vi "sender.vi"() -> ()   [LabVIEW 2009]
uses:
  Robot Status.ctl
  <vilib>/Platform/TimedLoop/XDataNode/XDataNode.xnode
  <vilib>/Platform/TimedLoop/XDataNode/loadlvalarms.vi
  <vilib>/Platform/TimedLoop/XDataNode/timing_clust.ctl
  <vilib>/Platform/TimedLoop/XDataNode/nitl_modes.ctl
  <vilib>/Platform/TimedLoop/XDataNode/wakeup.ctl
  UDP Lib/UDP Network Location.ctl
  cRIO/Functional Global Variables/Actions for FG's.ctl
  <vilib>/Platform/TimedLoop/XDataNode/XDNodeRunTimeDep.lvlib
panel:
  out "Status out":T1
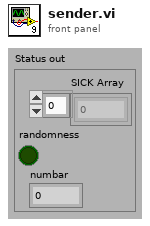
[diagram p1: front panel]
types:
  T1 = typedef "Robot Status.ctl" = cluster{"SICK Array":dbl[], "randomness":bool, "numbar":dbl}
  T2 = typedef "UDP Base.ctl" = cluster{"UDP Session":refnum<k16>, "UDP Socket Params":T3}
  T3 = typedef "UDP Socket Params.ctl" = cluster{"Local Port":u16, "Read Timeout":i32, "Write Timeout":i32}
  T4 = typedef "XDNodeRunTimeDep.lvlib/timing_clust.ctl" = cluster{"Expected End [f-1]":u64, "Actual End [f-1]":u64, "Finished Late? [f-1]":bool, "Expected End [i-1]":u64, "Actual End [i-1]":u64, "Finished Late? [i-1]":bool, "Expected Start [i]":u64, "Actual Start [i]":u64, "Expected Start [f]":u64, "Actual Start [f]":u64, "Source Name":string, "Structure Name":string, "Period":i64, "Deadline":i64, "Offset":i64, "Start":i64, "Priority":i32, "Timeout":i32, "Mode":T5, "Wakeup Reason":T6, "Error":errorcluster, "Source Type":string, "Secondary Source Type":string, "Global End Time":u64, "Global Start Time":u64, "Frame Duration":u64, "Iteration Duration":u64, "Assigned CPU":i32, "I/O Scan Engine Mode":u32}
  T5 = typedef "XDNodeRunTimeDep.lvlib/nitl_modes.ctl" = enum32{"No Change", "Process missed periods, maintain original phase", "Discard missed periods, maintain original phase", "Process missed periods, ignore original phase", "Discard missed periods, ignore original phase"}
  T6 = typedef "XDNodeRunTimeDep.lvlib/wakeup.ctl" = enum32{"Normal", "Aborted", "Asynchronous wakeup", "Timing source error", "Timed loop error", "Timeout"}
  T7 = typedef "UDP Network Location.ctl" = cluster{"IP Address":string, "Port":u16}
  T8 = typedef "Actions for FG's.ctl" = enum16{"Read", "Write"}
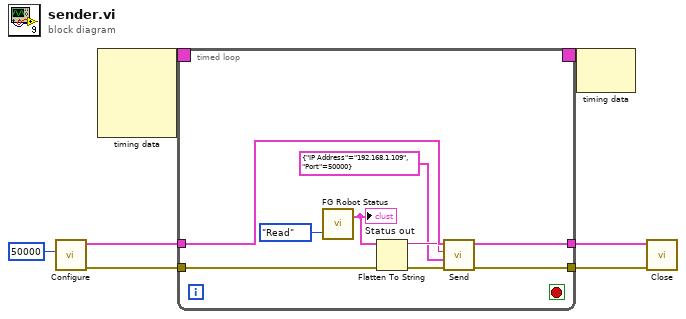
[diagram p0: block diagram]
diagram:
  n1 = call "Configure.vi"("Local Port"=u16 50000) -> ("error out"=w2:errorcluster, "UDP Base out"=w3:T2)  [unwired: 9 in]
  n2 = node-c288() -> (w7:T4)  [unwired: 4 in]
  n3 = timed-loop {
    timing: w7 -> [_]
    timing-out: [_] -> w6
    tunnel: [w15] -> w5
    tunnel: [w14] -> w4
    tunnel: w3 -> [w13]
    tunnel: w2 -> [w10]
    stop <- _ stop-if-true
    n4 = call "FG Robot Status.vi"("FG Action"=Actions_for_FG's."Read") -> ("Status out"=w12:T1)  [unwired: 2 in]
    "Status out" <- w12
    n5 = Flatten To String(anything=w12, error in (no error)=w10) -> (data string=w11:string, error out=w9:errorcluster)  [unwired: 2 in, 1 out]
    n6 = call "Send.vi"("error in (no error)"=w9, "Destination Location"=T7 {"IP Address"="192.168.1.109", "Port"=50000}, "Send Data"=w11, "UDP Base in"=w13) -> ("error out"=w14:errorcluster, "UDP Base out"=w15:T2)  [unwired: 5 in, 1 out]
  }
  n7 = node-c288(w6) -> ()  [unwired: 1 out]
  n8 = call "Close.vi"("error in (no error)"=w4, "Cluster of class private data"=w5) -> ()  [unwired: 9 in, 1 out]
